vi "OpenLoop_TCrane.vi"() -> ()   [LabVIEW 2009]
uses:
  Instance           2 23Saved   OpenLoop_TCrane .vi
  Instance           3 23Saved   OpenLoop_TCrane .vi
  Instance           4 23Saved   OpenLoop_TCrane .vi
  Instance           5 23Saved   OpenLoop_TCrane .vi
  RTDACUSB_TCrane.dll
panel:
  out "RESET value":dbl format="%#.12g"
  in  "Reset encoders":bool
  out "XY Graph":cluster{"Y":dbl[], "Y":dbl[]}[](graph)
  out "Z displacement chart":dbl(graph)
  out "Y displacement chart":dbl(graph)
  out "X displacement chart":dbl(graph)
  out "Z-axis limit flag":bool
  out "T-angle limit flag":bool
  out "X-axis limit flag":bool
  out "Z-axis therm flag":bool
  out "T-angle therm flag":bool
  out "X-axis therm flag":bool
  in  "Stop motors":bool
  in  "Therm flags":T1(radio)
  in  "Limit flags":T2(radio)
  out "Encoder Beta":dbl format="%#.12g"
  out "Encoder Alfa":dbl format="%#.12g"
  out "Encoder Z":dbl format="%#.12g"
  out "Encoder Theta":dbl format="%#.12g"
  out "Numeric 3":dbl
  out "Z - Motor On/Off":bool
  in  "Z-Motor On/Off":bool
  in  "Z-axis control":dbl(slide) scale=-1.0..1.0
  out "Numeric 2":dbl
  out "Theta - Motor On/Off":bool
  in  "T-Motor On/Off":bool
  in  "Theta-angle control":dbl(slide) scale=-1.0..1.0
  out "Last error":string
  out "Logic version":dbl
  out "No of detected boards":dbl
  out "Numeric":dbl
  out "X - Motor On/Off":bool
  in  "X-Motor On/Off":bool
  in  "X-axis control":dbl(slide) scale=-1.0..1.0
  out "Encoder X":dbl format="%#.12g"
  out "Counter pulses":dbl format="%#.12g"
  out "Sample time [ms]":dbl format="%#.12g"
  out "Waveform Chart":i32(graph)
  in  "stop 2":bool
  # "Tower Crane: Manual setup"
  # "RT-DAC/USB status"
  # "Tower Crane motor control"
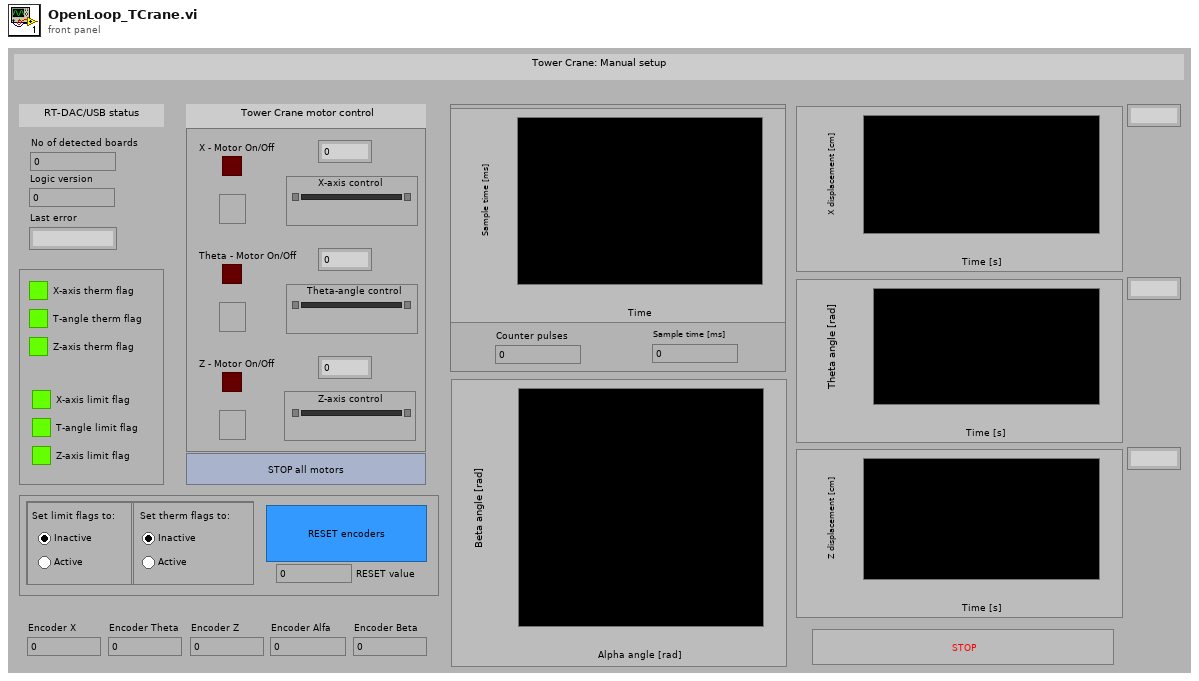
[diagram p1: front panel]
types:
  T1 = enum32{"Set therm flags to:", "Radio Selection 2"}
  T2 = enum32{"Set limit flags to:", "Radio Selection 2"}
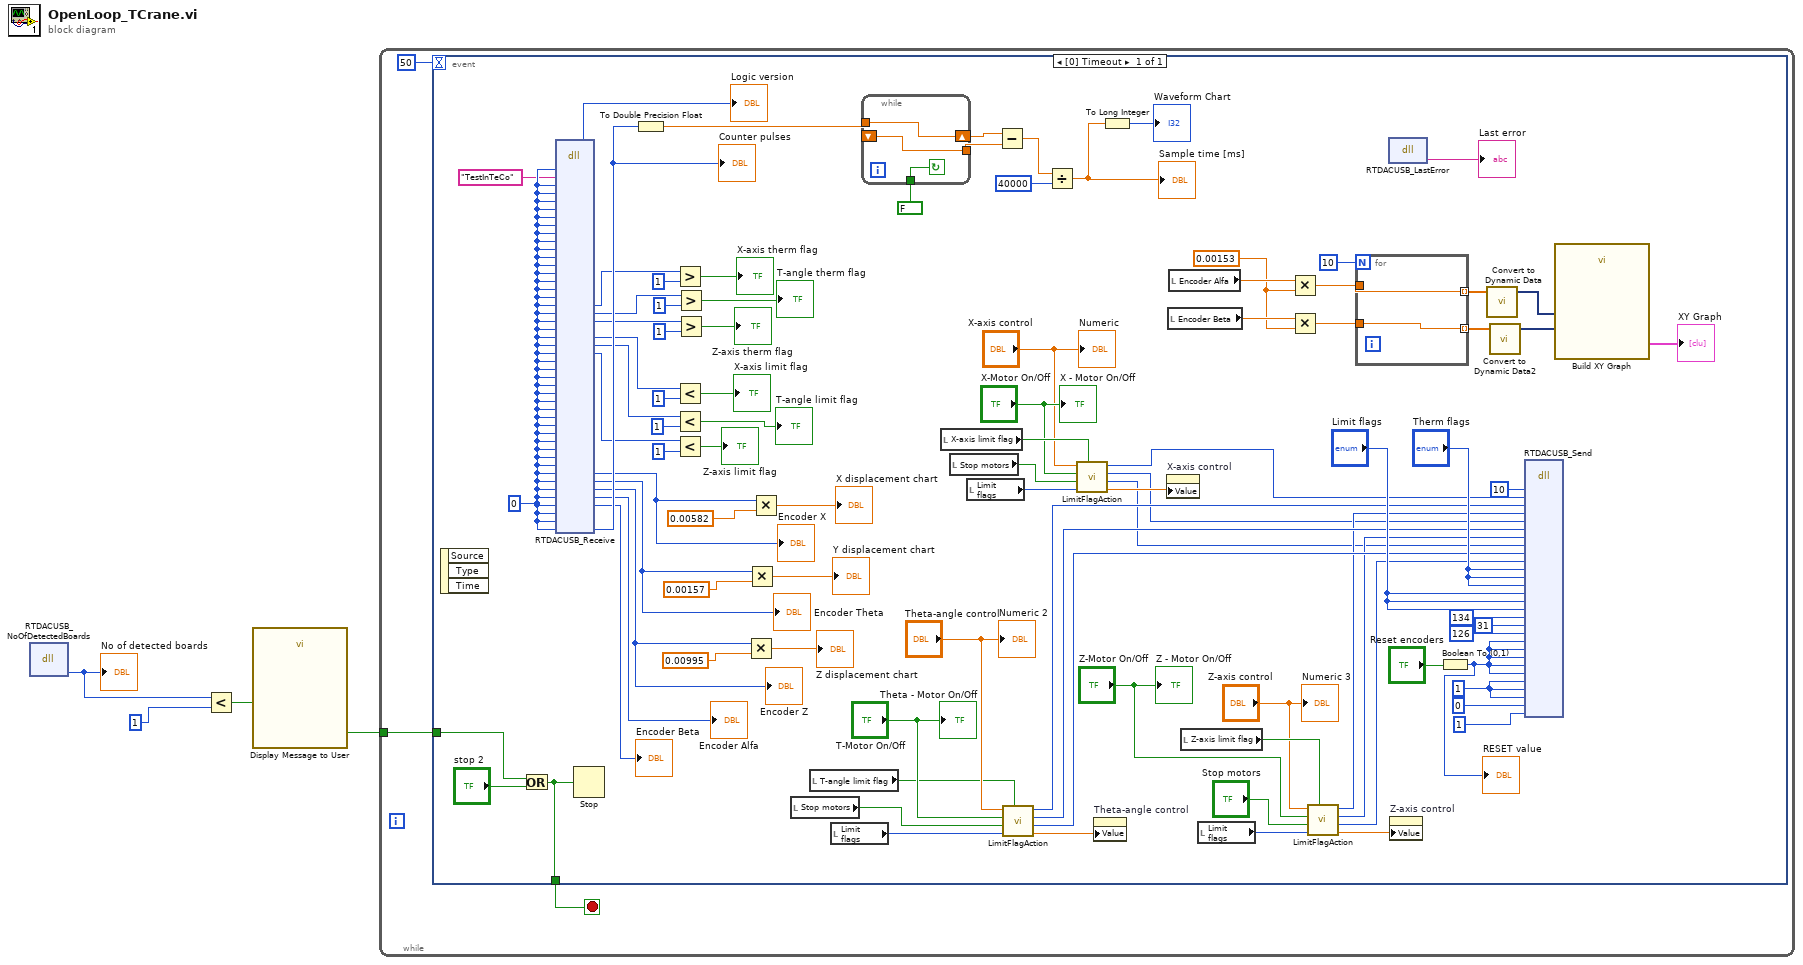
[diagram p0: block diagram]
diagram:
  n1 = dll-call lib="\\\\afs\\md.kth.se/ee/prj/regler_prj/2010/cranecont/Project-Data/Initial-VI/RTDACUSB_TCrane.dll" fn="RTDACUSB_NoOfDetectedBoards" ("PlxApi.dll:PlxBusIopWrite")() -> ("pNoOfDetectedBoards"=w4:i32)  [unwired: 5 in, 2 out]
  "No of detected boards" <- w4
  n2 = Less?(x=w4, y=1) -> (x < y?=w3:bool)
  n3 = call "Display Message to User"("Enable"=w3) -> ("OK"=w1:bool)  [unwired: 9 in, 1 out]
  n4 = while {
    tunnel: w1 -> [w5]
    stop <- w6 stop-if-true
    n5 = event shown="[0] Timeout" {
      selector: _ -> [_]
      dyn-events: _ -> [_]
      timeout: 50 -> [_]
      tunnel: [w78] -> w6
      tunnel: w5 -> [w80]
      event [0] Timeout {
        w39 = 0.00153
        w87 = 1
        w92 = 0
        n6 = event-data() -> ()  [unwired: 1 in, 3 out]
        n7 = Or(x=w80, y="stop 2") -> (x .or. y?=w78:bool)
        n8 = dll-call lib="\\\\afs\\md.kth.se/ee/prj/regler_prj/2010/cranecont/Project-Data/Initial-VI/RTDACUSB_TCrane.dll" fn="RTDACUSB_Receive" ("PlxApi.dll:PlxBusIopWrite")("pLogicVersion"=w92, "pApplicationName"="TestInTeCo", "pCN1Direction"=w92, "pCN1Input"=w92, "pPWMDivider"=w92, "pPWMWidth0"=w92, "pPWMWidth1"=w92, "pPWMWidth2"=w92, "pPWMDir0"=w92, "pPWMDir1"=w92, "pPWMDir2"=w92, "pPWMBrake0"=w92, "pPWMBrake1"=w92, "pPWMBrake2"=w92, "pPWMTherm0"=w92, "pPWMTherm1"=w92, "pPWMTherm2"=w92, "pPWMThermFlag0"=w92, "pPWMThermFlag1"=w92, "pPWMThermFlag2"=w92, "pNOFlag"=w92, "pLimitActive0"=w92, "pLimitActive1"=w92, "pLimitActive2"=w92, "pLimitFlag0"=w92, "pLimitFlag1"=w92, "pLimitFlag2"=w92, "pLimit0"=w92, "pLimit1"=w92, "pLimit2"=w92, "pEncoderReset0"=w92, "pEncoderReset1"=w92, "pEncoderReset2"=w92, "pEncoderReset3"=w92, "pEncoderReset4"=w92, "pEncoderAutoResetFlag0"=w92, "pEncoderAutoResetFlag1"=w92, "pEncoderAutoResetFlag2"=w92, "pEncoder0"=w92, "pEncoder1"=w92, "pEncoder2"=w92, "pEncoder3"=w92, "pEncoder4"=w92, "pTmrCnt0_Reset"=w92, "pTmrCnt0_Mode"=w92, "pTmrCnt0_Counter"=w92) -> ("pLogicVersion"=→"Logic version":u32, "pPWMThermFlag0"=w66:u32, "pPWMThermFlag1"=w67:u32, "pPWMThermFlag2"=w68:u32, "pLimitActive0"=w38:u32, "pLimitActive1"=w36:u32, "pLimitActive2"=w37:u32, "pEncoder0"=w52:i32, "pEncoder1"=w48:i32, "pEncoder2"=w44:i32, "pEncoder3"=→"Encoder Alfa":i32, "pEncoder4"=→"Encoder Beta":i32, "pTmrCnt0_Counter"=w93:u32)  [unwired: 37 in, 2 out]
        "Counter pulses" <- w93
        "Encoder X" <- w52
        "Encoder Theta" <- w48
        "Encoder Z" <- w44
        n9 = Stop(stop? (T)=w78) -> ()
        n10 = To Double Precision Float(number=w93) -> (double precision float=w101:dbl)
        n11 = Greater?(x=w66, y=1) -> (0:→"X-axis therm flag":bool)
        n12 = Less?(x=w38, y=1) -> (x < y?=→"X-axis limit flag":bool)
        n13 = Less?(x=w36, y=1) -> (x < y?=→"T-angle limit flag":bool)
        n14 = Less?(x=w37, y=1) -> (x < y?=→"Z-axis limit flag":bool)
        n15 = Greater?(x=w67, y=1) -> (0:→"T-angle therm flag":bool)
        n16 = Greater?(x=w68, y=1) -> (0:→"Z-axis therm flag":bool)
        n17 = Multiply(x=w44, y=0.00995) -> (x*y=→"Z displacement chart":dbl)
        n18 = Multiply(x=w48, y=0.00157) -> (x*y=→"Y displacement chart":dbl)
        n19 = Multiply(x=w52, y=0.00582) -> (x*y=→"X displacement chart":dbl)
        n20 = local read "Stop motors"() -> (w33:bool)
        n21 = local read "T-angle limit flag"() -> (w29:bool)
        n22 = local read "Limit flags"() -> (w34:T2)
        n23 = while {
          shift-right: [w106] -> w100
          shift-left: _ -> [w105]
          tunnel: w101 -> [w106]
          tunnel: [w105] -> w99
          tunnel: FALSE -> [w104]
          stop <- w104 continue-if-true
        }
        n24 = local read "X-axis limit flag"() -> (w13:bool)
        n25 = local read "Stop motors"() -> (w14:bool)
        n26 = local read "Limit flags"() -> (w15:T2)
        n27 = Subtract(x=w100, y=w99) -> (x-y=w98:dbl)
        n28 = call "LimitFlagAction.vi"("Axis limit flag"=w29, "Global limit flag active"=w34, "Stop motors global"=w33, "Stop motor local"="T-Motor On/Off", "Axis control signal"="Theta-angle control") -> ("Slider control"=w32:dbl, "PWM Brake"=w28:u32, "PWM Direction"=w27:u32, "PWM width"=w26:u32)
        n29 = Divide(x=w98, y=40000) -> (x/y=w95:dbl)
        "Sample time [ms]" <- w95
        n30 = call "LimitFlagAction.vi"("Axis limit flag"=w13, "Global limit flag active"=w15, "Stop motors global"=w14, "Stop motor local"="X-Motor On/Off", "Axis control signal"="X-axis control") -> ("Slider control"=w16:dbl, "PWM Brake"=w10:u32, "PWM Direction"=w9:u32, "PWM width"=w8:u32)
        n31 = property on="Theta-angle control" class="Slide (strict)"("Value"=w32) -> ()  [unwired: 2 in, 2 out]
        n32 = To Long Integer(number=w95) -> (32bit integer=→"Waveform Chart":i32)
        n33 = property on="X-axis control" class="Slide (strict)"("Value"=w16) -> ()  [unwired: 2 in, 2 out]
        n34 = local read "Encoder Beta"() -> (w40:dbl)
        n35 = local read "Encoder Alfa"() -> (w41:dbl)
        n36 = local read "Z-axis limit flag"() -> (w19:bool)
        n37 = local read "Limit flags"() -> (w21:T2)
        n38 = Multiply(x=w41, y=w39) -> (x*y=w43:dbl)
        n39 = Multiply(x=w40, y=w39) -> (x*y=w42:dbl)
        n40 = call "LimitFlagAction.vi"("Axis limit flag"=w19, "Global limit flag active"=w21, "Stop motors global"="Stop motors", "Stop motor local"="Z-Motor On/Off", "Axis control signal"="Z-axis control") -> ("Slider control"=w25:dbl, "PWM Brake"=w24:u32, "PWM Direction"=w23:u32, "PWM width"=w22:u32)
        n41 = for {
          N: 10 -> [_]
          tunnel: w42 -> [w102]
          tunnel: w43 -> [w103]
          tunnel: [w103] -> w56 mode=indexing
          tunnel: [w102] -> w55 mode=indexing
        }
        n42 = dll-call lib="\\\\afs\\md.kth.se/ee/prj/regler_prj/2010/cranecont/Project-Data/Initial-VI/RTDACUSB_TCrane.dll" fn="RTDACUSB_LastError" ("PlxApi.dll:PlxBusIopWrite")() -> ("dsrp"=→"Last error":string)  [unwired: 3 in, 2 out]
        n43 = property on="Z-axis control" class="Slide (strict)"("Value"=w25) -> ()  [unwired: 2 in, 2 out]
        n44 = Boolean To (0,1)(Boolean="Reset encoders") -> (0, 1=w53:i16)
        "RESET value" <- w53
        n45 = call "Convert to Dynamic Data"("Array"=w56) -> ("Dynamic Data Type"=w57:dynamicdata)  [unwired: 3 in]
        n46 = call "Convert to Dynamic Data2"("Array"=w55) -> ("Dynamic Data Type"=w59:dynamicdata)  [unwired: 3 in]
        n47 = dll-call lib="\\\\afs\\md.kth.se/ee/prj/regler_prj/2010/cranecont/Project-Data/Initial-VI/RTDACUSB_TCrane.dll" fn="RTDACUSB_Send" ("PlxApi.dll:PlxBusIopWrite")("PWMDivider"=10, "PWMWidth0"=w8, "PWMWidth1"=w26, "PWMWidth2"=w22, "PWMDir0"=w9, "PWMDir1"=w27, "PWMDir2"=w23, "PWMBrake0"=w10, "PWMBrake1"=w28, "PWMBrake2"=w24, "PWMThermFlag0"="Therm flags", "PWMThermFlag1"="Therm flags", "PWMThermFlag2"="Therm flags", "LimitFlag0"="Limit flags", "LimitFlag1"="Limit flags", "LimitFlag2"="Limit flags", "Limit0"=134, "Limit1"=31, "Limit2"=126, "EncoderReset0"=w53, "EncoderReset1"=w53, "EncoderReset2"=w53, "EncoderReset3"=w53, "EncoderReset4"=w53, "EncoderAutoResetFlag0"=w87, "EncoderAutoResetFlag1"=w87, "EncoderAutoResetFlag2"=w87, "TmrCnt0_Reset"=0, "TmrCnt0_Mode"=1) -> ()  [unwired: 33 in, 2 out]
        n48 = call "Build XY Graph"("Y Input"=w59, "X Input"=w57) -> ("XY Graph"=→"XY Graph":cluster{"Y":dbl[], "Y":dbl[]}[])  [unwired: 8 in, 1 out]
        "X - Motor On/Off" <- "X-Motor On/Off"
        "Numeric" <- "X-axis control"
        "Theta - Motor On/Off" <- "T-Motor On/Off"
        "Numeric 2" <- "Theta-angle control"
        "Z - Motor On/Off" <- "Z-Motor On/Off"
        "Numeric 3" <- "Z-axis control"
      }
    }
  }
